vi "Set Run Number.vi"(10 "run number":i32, 11 "AD* in":refnum<class "NI_Robotics_AnytimeDStar.lvclass">) -> (3 "AD* out":refnum<class "NI_Robotics_AnytimeDStar.lvclass">)   [LabVIEW 2017, in "NI_Robotics_AnytimeDStar.lvclass"]
uses:
  <vilib>/robotics/Navigation/Anytime D Star/NI_Robotics_AnytimeDStar.lvclass
  <vilib>/robotics/Navigation/Anytime D Star/NI_Robotics_AnytimeDStar.lvclass/NI_Robotics_AnytimeDStar.ctl
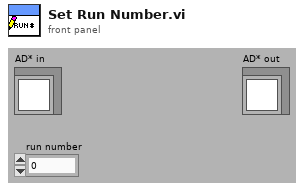
[diagram p1: front panel]
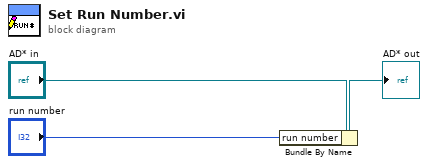
[diagram p0: block diagram]
diagram:
  n1 = Bundle By Name(cluster="AD* in", "run number"="run number") -> (→"AD* out":refnum<class "NI_Robotics_AnytimeDStar.lvclass">)
